vi "Build Folder Tree.vi"(11 "Library":refnum<vi>) -> (3 "Folder Tree":T1[](array[typedef]))   [LabVIEW 2018, in "LVClassByRef.lvlib"]
uses:
  <resource>/Framework/Providers/LVClassByRef/LVClassByRef.lvlib
  <resource>/Framework/Providers/LVClassByRef/Folder Item.ctl
  <resource>/Framework/Providers/LVClassByRef/Tree Item.ctl
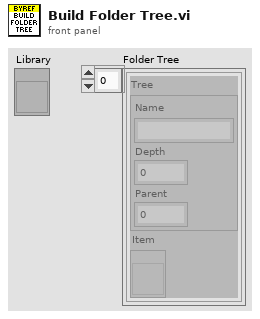
[diagram p1: front panel]
types:
  T1 = typedef "LVClassByRef.lvlib/Folder Item.ctl" = cluster{"Tree":T2, "Item":refnum<vi>}
  T2 = typedef "LVClassByRef.lvlib/Tree Item.ctl" = cluster{"Name":string, "Depth":i32, "Parent":i32}
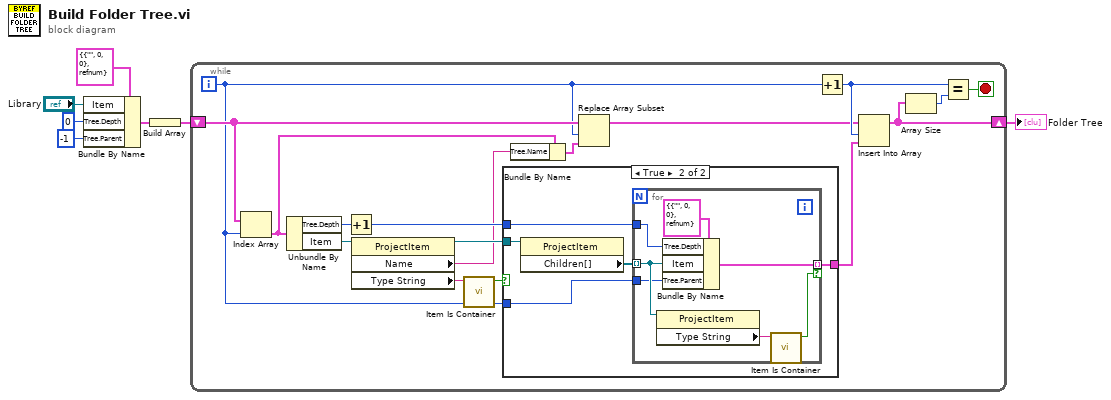
[diagram p0: block diagram]
diagram:
  n1 = Bundle By Name(cluster=T1 {"Tree"={"Name"="", "Depth"=0, "Parent"=0}, "Item"=refnum} ("Folder Item"), "Item"="Library", "Tree.Depth"=0 ("Depth"), "Tree.Parent"=-1) -> (w5:T1)
  n2 = Build Array(w5) -> (w4:T1[])
  n3 = while {
    shift-right: [w20] -> w3
    shift-left: w4 -> [w21]
    i -> [w8]
    stop <- w18 stop-if-true
    n4 = Index Array(array=w21, index=w8) -> (element=w14:T1)
    n5 = Unbundle By Name(w14) -> ("Tree.Depth"=w24:i32, "Item"=w23:refnum<vi>)
    n6 = Increment(x=w24) -> (x+1=w16:i32)
    n7 = property class="ProjectItem"(reference=w23) -> (reference out=w17:refnum<vi>, "Name"=w13:string, "Type String"=w10:string)  [unwired: 1 in, 1 out]
    n8 = call <resource>:"Item Is Container.vi"("Type String"=w10) -> ("Container?"=w9:bool)  [unwired: 10 in]
    n9 = case shown="True" w9 {
      tunnel: w17 -> [_ w29]
      tunnel: w16 -> [_ w28]
      tunnel: [_ w27] -> w11
      tunnel: w8 -> [_ w25]
      frame False {
      }
      frame True {
        n10 = property class="ProjectItem"(reference=w29) -> ("Children[]"=w26:refnum<vi>[])  [unwired: 1 in, 2 out]
        n11 = for {
          tunnel: w26 -> [w33] mode=indexing
          tunnel: w28 -> [w35]
          tunnel: [w34] -> w27 mode=indexing if=w31
          tunnel: w25 -> [w30]
          n12 = property class="ProjectItem"(reference=w33) -> ("Type String"=w32:string)  [unwired: 1 in, 2 out]
          n13 = Bundle By Name(cluster=T1 {"Tree"={"Name"="", "Depth"=0, "Parent"=0}, "Item"=refnum} ("Folder Item"), "Tree.Depth"=w35, "Item"=w33, "Tree.Parent"=w30) -> (w34:T1)
          n14 = call <resource>:"Item Is Container.vi"("Type String"=w32) -> ("Container?"=w31:bool)  [unwired: 10 in]
        }
      }
    }
    n15 = Bundle By Name(cluster=w14, "Tree.Name"=w13) -> (w12:T1)
    n16 = Replace Array Subset(array=w21, new element=w12, index=w8) -> (w15:T1[])
    n17 = Increment(x=w8) -> (x+1=w19:i32)
    n18 = Insert Into Array(array=w15, index=w19, new element=w11) -> (w20:T1[])
    n19 = Array Size(array=w20) -> (size(s)=w22:i32)
    n20 = Equal?(x=w19, y=w22) -> (x = y?=w18:bool)
  }
  "Folder Tree" <- w3
